vi "IndexLastActiveNeuron.vi"(11 "Neurons":refnum<class "Neuron.lvclass">[](array[class])) -> (3 "Last Neuron":i32)   [LabVIEW 2013, in "Neuron.lvclass"]
doc: "This Vi returns the index of the last neuron active in the network"
uses:
  Neuron/Neuron.lvclass
  Neuron/Neuron.lvclass/Neuron.ctl
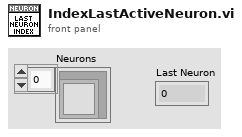
[diagram p1: front panel]
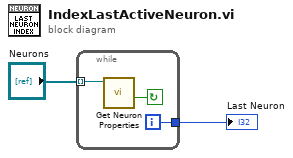
[diagram p0: block diagram]
diagram:
  n1 = while {
    tunnel: "Neurons" -> [w5] mode=indexing
    tunnel: [w4] -> w1
    i -> [w4]
    stop <- w3 continue-if-true
    n2 = call "Get Neuron Properties.vi"("Neuron in"=w5) -> ("Active"=w3:bool)  [unwired: 5 in, 5 out]
  }
  "Last Neuron" <- w1
